vi "Main.vi"() -> ()   [LabVIEW 2017]
uses:
  Controls/W_Testi_Control.ctl
panel:
  in  "btnDivide":bool
  in  "btnMultiply":bool
  in  "btnStop":bool
  in  "Cluster":T1
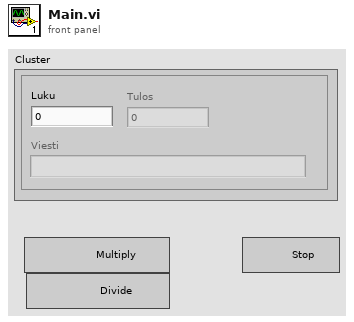
[diagram p1: front panel]
types:
  T1 = typedef "W_Testi_Control.ctl" = cluster{"Luku":dbl, "Tulos":dbl, "Viesti":string}
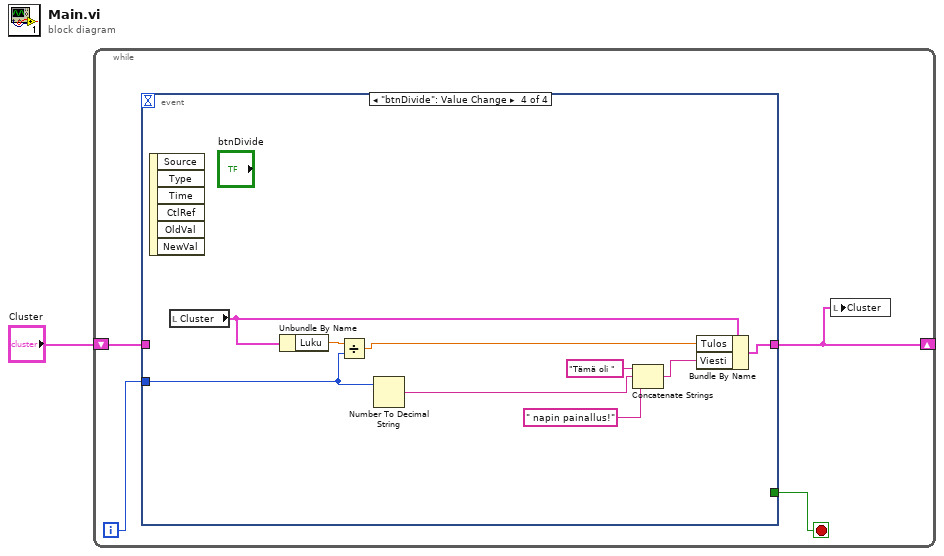
[diagram p0: block diagram]
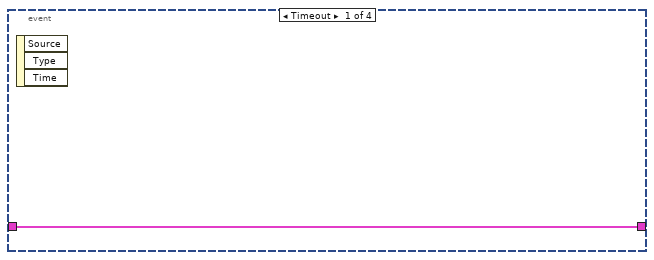
[diagram p2: hidden frame]
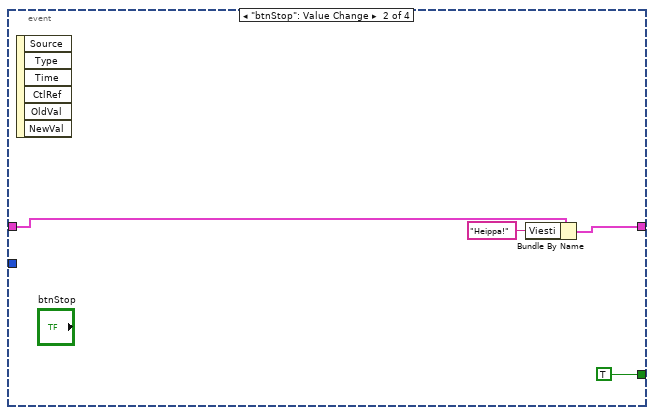
[diagram p3: hidden frame]
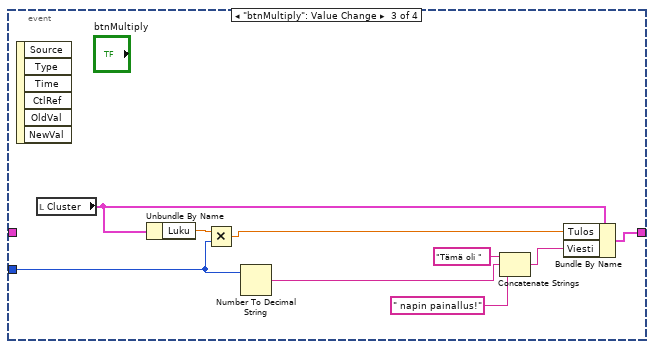
[diagram p4: hidden frame]
diagram:
  n1 = while {
    shift-right: [w3] -> _
    shift-left: "Cluster" -> [w4]
    i -> [w2]
    stop <- w5 stop-if-true
    n2 = event shown="[3] \"btnDivide\": Value Change" {
      selector: _ -> [_ _ _ _]
      dyn-events: _ -> [_ _ _ _]
      timeout: _ -> [_ _ _ _]
      tunnel: [_ TRUE _ _] -> w5
      tunnel: w4 -> [w6 w9 _ _]
      tunnel: [w6 w8 w19 w28] -> w3
      tunnel: w2 -> [_ _ w14 w23]
      event Timeout {
        n3 = event-data() -> ()  [unwired: 1 in, 3 out]
      }
      event "btnStop": Value Change {
        n4 = event-data() -> ()  [unwired: 1 in, 6 out]
        n5 = Bundle By Name(cluster=w9, "Viesti"="Heippa!") -> (w8:T1)
      }
      event "btnMultiply": Value Change {
        n6 = event-data() -> ()  [unwired: 1 in, 6 out]
        n7 = local read "Cluster"() -> (w11:T1)
        n8 = Unbundle By Name(w11) -> ("Luku"=w18:dbl)
        n9 = Multiply(x=w18, y=w14) -> (x*y=w17:dbl)
        n10 = Number To Decimal String(number=w14) -> (decimal integer string=w13:string)  [unwired: 1 in]
        n11 = Concatenate Strings("Tämä oli " ("string"), w13, " napin painallus!" ("string")) -> (w16:string)
        n12 = Bundle By Name(cluster=w11, "Tulos"=w17, "Viesti"=w16) -> (w19:T1)
      }
      event "btnDivide": Value Change {
        n13 = event-data() -> ()  [unwired: 1 in, 6 out]
        n14 = local read "Cluster"() -> (w20:T1)
        n15 = Unbundle By Name(w20) -> ("Luku"=w27:dbl)
        n16 = Divide(x=w27, y=w23) -> (x/y=w26:dbl)
        n17 = Number To Decimal String(number=w23) -> (decimal integer string=w22:string)  [unwired: 1 in]
        n18 = Concatenate Strings("Tämä oli " ("string"), w22, " napin painallus!" ("string")) -> (w25:string)
        n19 = Bundle By Name(cluster=w20, "Tulos"=w26, "Viesti"=w25) -> (w28:T1)
      }
    }
    n20 = local write "Cluster"(w3) -> ()
  }
